vi "有效状态.vi"(4 "脉冲选择":u8, 5 "串口号":refnum<visa-resource-name>) -> (1 "应答":string)   [LabVIEW 2014]
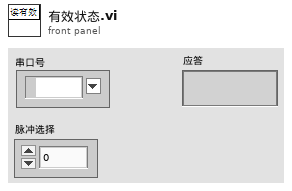
[diagram p1: front panel]
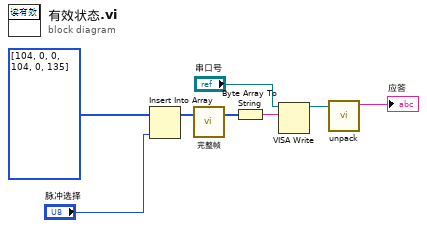
[diagram p0: block diagram]
diagram:
  n1 = Insert Into Array(array=u8[] [104, 0, 0, 104, 0, 135], new element="脉冲选择") -> (w4:u8[])  [unwired: 1 in]
  n2 = call "完整帧.vi"("不完整帧"=w4) -> ("完整帧"=w8:u8[])  [unwired: 2 in]
  n3 = Byte Array To String(unsigned byte array=w8) -> (string=w7:string)
  n4 = VISA Write(VISA resource name="串口号", write buffer=w7) -> (VISA resource name out=w2:refnum<visa-resource-name>)  [unwired: 1 in, 2 out]
  n5 = call "unpack.vi"("串口号输入"=w2) -> ("应答"=→"应答":string)  [unwired: 5 in, 1 out]
